vi "Send Set Result Settings.vi"(7 "Message Priority (Normal)":T1=enum."Normal", 8 "error in (no error)":errorcluster, 10 "Analyze Results":refnum<class "Analyze Results Base.lvclass">, 11 "Message Enqueuer":refnum<class "Message Enqueuer.lvclass">) -> (0 "error out":errorcluster, 3 "Message Enqueuer out":refnum<class "Message Enqueuer.lvclass">)   [LabVIEW 2020, in "HIJ Vision Application.lvlib" / "Set Result Settings Msg.lvclass"]
doc: "This VI sends the message to an actor."
uses:
  Set Result Settings Msg.lvclass
  Set Result Settings Msg.lvclass/Set Result Settings Msg.ctl
  <vilib>/ActorFramework/Message Enqueuer/Message Enqueuer.lvclass
  C:/Program Files (x86)/National Instruments/LabVIEW 2020/vi.lib/ActorFramework/Message/Message.lvclass
  C:/Users/AlexK/work/LabVIEW Programme/POLARIS-AS-3-Cams/Submodules/HIJ Vision/Application Base Actors/HIJ Vision Application/HIJ Vision Application Messages/Set Result Settings Msg/Set Result Settings Msg.lvclass
  <vilib>/ActorFramework/Message Enqueuer/Message Priority.ctl
  Analyze/Results and Overlays/Results Base/Analyze Results Base.lvclass
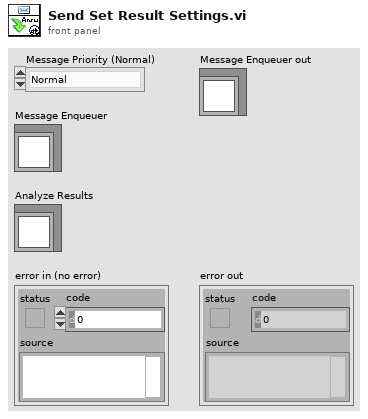
[diagram p1: front panel]
types:
  T1 = typedef "Actor Framework.lvlib/Message Enqueuer.lvclass/Message Priority.ctl" = enum16{"Low", "Normal", "High"}
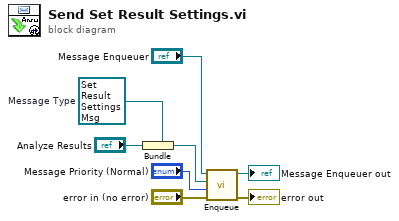
[diagram p0: block diagram]
diagram:
  w5 = refnum<class "Set Result Settings Msg.lvclass"> refnum  # Message Type
  n1 = Bundle(cluster=w5, "Analyze Results") -> (w4:refnum<class "Set Result Settings Msg.lvclass">)
  n2 = call <vilib>:"Enqueue.vi"("error in (no error)"="error in (no error)", "Message Priority (Normal)"="Message Priority (Normal)", "Message"=w4, "Message Enqueuer in"="Message Enqueuer") -> ("error out"=→"error out":errorcluster, "Message Enqueuer in"=→"Message Enqueuer out":refnum<class "Message Enqueuer.lvclass">)  [unwired: 6 in]
